vi "Convert State For Save.vi"(2 "Container State":T1, 3 "Display State":T2) -> (1 "Display State To Save":variant)   [LabVIEW 2020, in "3D Surface.xctl"]
uses:
  3D Surface.xctl
  State.ctl
  3D Surface.lvclass
  e:/builds/penguin/labview/branches/2020/dev/dist/vi.lib/Math Plots/3D Math Plots/3D Plot/3D Plot/3D Plot.lvclass
  3DMathPlot Ctrl Act Queue.ctl
  3DMathPlot Ctrl Act Cluster.ctl
  3DMathPlot State Class.ctl
  Container State.ctl
  3D Plot.lvclass
  XControlSupport.lvlib
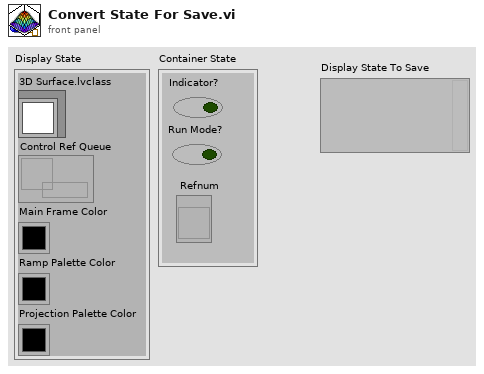
[diagram p1: front panel]
types:
  T1 = typedef "XControlSupport.lvlib/Container State.ctl" = cluster{"Indicator?":bool, "Run Mode?":bool, " Refnum":refnum<vi>}
  T2 = typedef "3D Surface.xctl/State.ctl" = cluster{"3D Surface.lvclass":refnum<class "3D Surface.lvclass">, "Control Ref Queue":T3, "Main Frame Color":u32, "Ramp Palette Color":u32, "Projection Palette Color":u32}
  T3 = typedef "3DMathPlot Ctrl Act Queue.ctl" = refnum<queue>
  T4 = enum32{"Towards X-Y Plane", "Towards X-Z Plane", "Towards Y-Z Plane", "User Defined"}
  T5 = typedef "3DMathPlot Ctrl Act Cluster.ctl" = cluster{"3D Picture Control":refnum<vi>, "Render Window Refnum":refnum<vi>, "XY Graph":refnum<vi>, "Intensity Graph":refnum<vi>, "Color Legend Palette":refnum<vi>, "Projection Palette":refnum<vi>, "XControl  Ref":refnum<vi>, "Facade Ref":refnum<vi>, "Export Image Ref":refnum<vi>, "Clear Data Flag":bool, "Display State Change Class":T6}
  T6 = typedef "3DMathPlot State Class.ctl" = enum16{"Update All Objects (Undo)", "Update Light Object Only", "Update Axis Object Only", "Update Plot Object Only", "Update Cursor Object Only", "Update Axis Plot Cursor Objects", "No Update"}
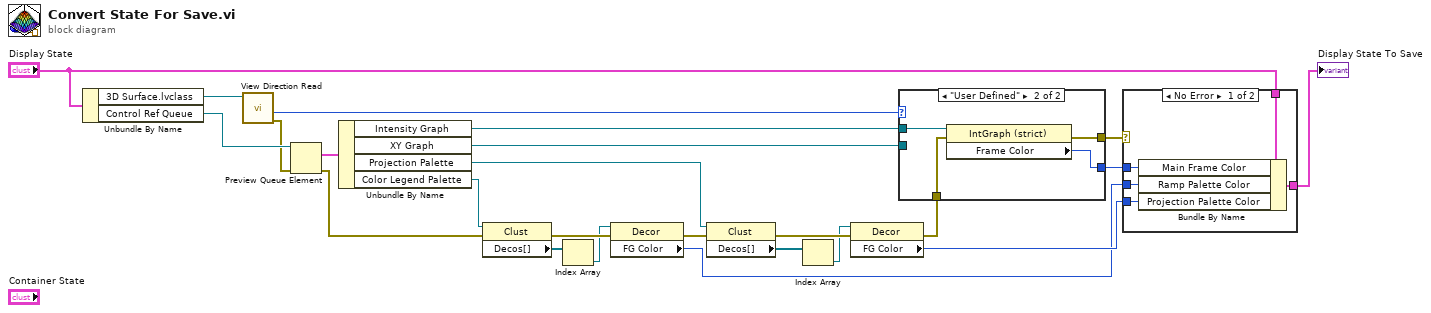
[diagram p0: block diagram]
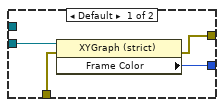
[diagram p3: hidden frame]
diagram:
  n1 = Unbundle By Name("Display State") -> ("3D Surface.lvclass"=w5:refnum<class "3D Surface.lvclass">, "Control Ref Queue"=w22:T3)
  n2 = call "View Direction Read.vi"("3D Plot.lvclass in"=w5) -> ("error out"=w2:errorcluster, "Value"=w4:T4)  [unwired: 8 in, 1 out]
  n3 = Preview Queue Element(queue=w22, error in (no error)=w2) -> (element=w21:T5, error out=w6:errorcluster)  [unwired: 3 out]
  n4 = Unbundle By Name(w21) -> ("Intensity Graph"=w3:refnum<vi>, "XY Graph"=w10:refnum<vi>, "Projection Palette"=w13:refnum<vi>, "Color Legend Palette"=w8:refnum<vi>)
  n5 = property class="Clust"(reference=w8, error in=w6) -> (error out=w18:errorcluster, "Decos[]"=w14:refnum<vi>[])  [unwired: 1 out]
  n6 = Index Array(array=w14) -> (element=w15:refnum<vi>)  [unwired: 1 in]
  n7 = property class="Decor"(reference=w15, error in=w18) -> (error out=w19:errorcluster, "FG Color"=w11:u32)  [unwired: 1 out]
  n8 = property class="Clust"(reference=w13, error in=w19) -> (error out=w20:errorcluster, "Decos[]"=w17:refnum<vi>[])  [unwired: 1 out]
  n9 = Index Array(array=w17) -> (element=w16:refnum<vi>)  [unwired: 1 in]
  n10 = property class="Decor"(reference=w16, error in=w20) -> (error out=w7:errorcluster, "FG Color"=w12:u32)  [unwired: 1 out]
  n11 = case shown="\"User Defined\"" w4 {
    tunnel: w10 -> [w28 _]
    tunnel: [w27 w30] -> w9
    tunnel: w7 -> [w26 w31]
    tunnel: w3 -> [_ w32]
    tunnel: [w25 w29] -> w1
    frame Default {
      n12 = property class="XYGraph (strict)"(reference=w28, error in=w26) -> (error out=w25:errorcluster, "Frame Color"=w27:u32)  [unwired: 1 out]
    }
    frame "User Defined" {
      n13 = property class="IntGraph (strict)"(reference=w32, error in=w31) -> (error out=w29:errorcluster, "Frame Color"=w30:u32)  [unwired: 1 out]
    }
  }
  n14 = case shown="No Error" w1 {
    tunnel: [w37 w38] -> w24
    tunnel: "Display State" -> [w36 w38]
    tunnel: w12 -> [w35 _]
    tunnel: w11 -> [w34 _]
    tunnel: w9 -> [w33 _]
    frame No Error {
      n15 = Bundle By Name(cluster=w36, "Main Frame Color"=w33, "Ramp Palette Color"=w34, "Projection Palette Color"=w35) -> (w37:T2)
    }
    frame Error {
    }
  }
  "Display State To Save" <- w24
